vi "Exemple_Model_Selection_GroupKFold_2.vi"() -> ()   [LabVIEW 2020]
uses:
  Objet/3 - Model selection and evaluation/Splitter/GroupKFold_2/GroupKFold_2.lvclass
panel:
  in  "Splitter en entrée":refnum<class "GroupKFold_2.lvclass">
  out "error out 2":errorcluster caption="sortie d'erreur"
  out "Out":T1={"train_index"=[[1.0, 2.0], [3.0, 4.0], [5.0, 6.0], [7.0, 8.0]], "test_index"=[[1.0, 2.0], [3.0, 4.0], [5.0, 6.0], [7.0, 8.0]]}
  out "Splitter en sortie":refnum<class "GroupKFold_2.lvclass">
  in  "n_splits":u8=2
  in  "In":cluster{"X":dbl[][], "y":dbl[], "groups":dbl[]}={"X"=[[1.0, 2.0], [3.0, 4.0], [5.0, 6.0], [7.0, 8.0]], "y"=[1.0, 2.0, 3.0, 4.0], "groups"=[]}
  in  "error in (no error)":errorcluster caption="entrée d'erreur (pas d'erreur)"
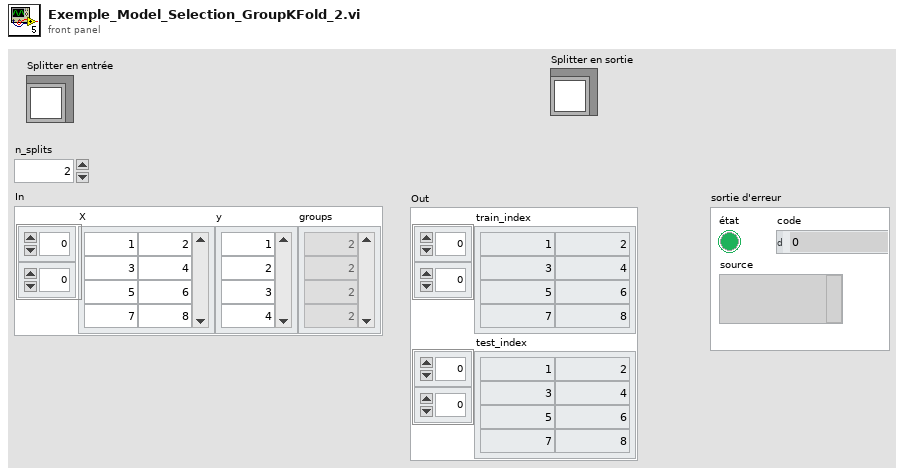
[diagram p1: front panel]
types:
  T1 = cluster{"train_index":dbl[][], "test_index":dbl[][]}
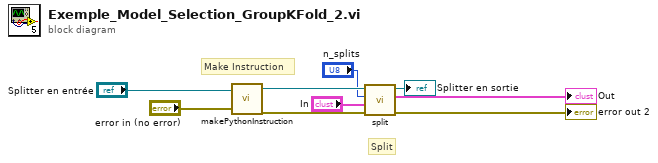
[diagram p0: block diagram]
diagram:
  # "Split"
  # "Make Instruction"
  n1 = call-dynamic "makePythonInstruction.vi"("error in (no error)"="error in (no error)", "Splitter en entrée"="Splitter en entrée") -> ("error out"=w7:errorcluster, "Splitter en sortie"=w8:refnum<class "GroupKFold_2.lvclass">)  [unwired: 8 in]
  n2 = call-dynamic "split.vi"("error in (no error) 2"=w7, "In"="In", "n_splits"="n_splits", "Splitter en entrée"=w8) -> ("error out 2"=→"error out 2":errorcluster, "Out"=→"Out":T1, "Splitter en sortie"=→"Splitter en sortie":refnum<class "GroupKFold_2.lvclass">)  [unwired: 5 in]
